vi "Header data_MClr.vi"(0 "base path":path=path "C:/", 1 "prompt (Create Folder)":string="logsController", 2 "file name":string, 5 "Error In":errorcluster) -> (14 "refnum out":refnum<file>, 19 "error out":errorcluster)   [LabVIEW 2018]
uses:
  Global textParse.vi
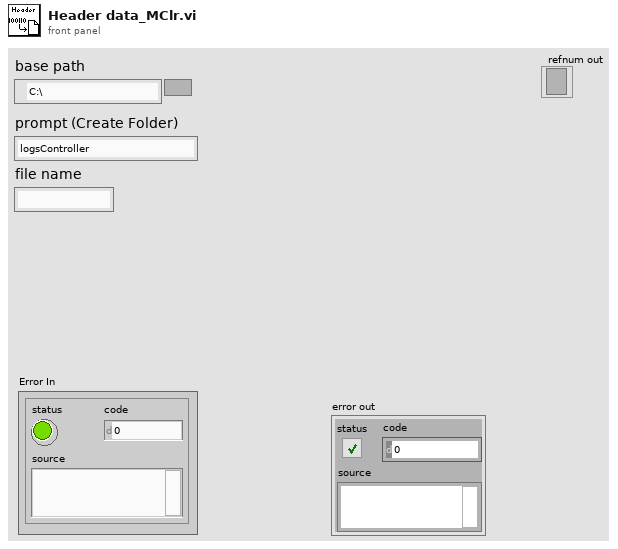
[diagram p1: front panel]
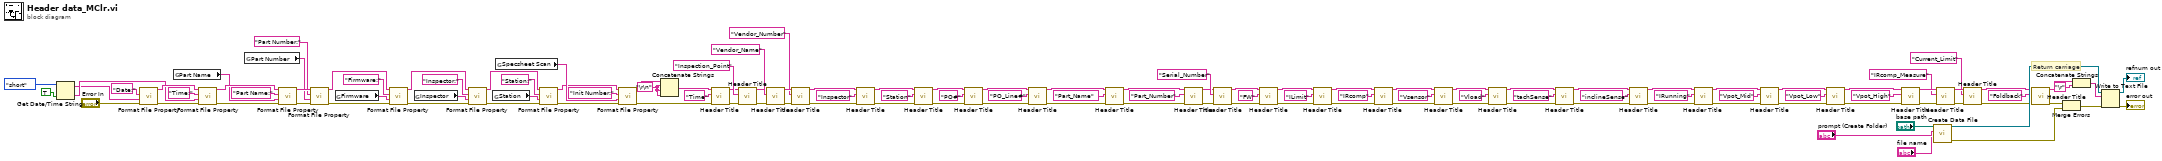
[diagram p0: block diagram]
diagram:
  w27 = "\r\n"
  # "Return carriage"
  n1 = Get Date/Time String(date format (0)=enum16{"short", "long", "abbreviated"}."short", want seconds? (F)=TRUE) -> (date string=w40:string, time string=w41:string)  [unwired: 1 in]
  n2 = call "Format File Property.vi"("Error In"="Error In", "File Property Value"=w40, "File Property Name"="Date:") -> ("Error Out"=w47:errorcluster, "String out"=w46:string)  [unwired: 7 in]
  n3 = global read "Global textParse.vi" "Part Name"() -> (w36:string)
  n4 = call "Format File Property.vi"("Error In"=w47, "File Property Value"=w41, "File Property Name"="Time:", "String in"=w46) -> ("Error Out"=w44:errorcluster, "String out"=w45:string)  [unwired: 6 in]
  n5 = global read "Global textParse.vi" "Part Number"() -> (w35:string)
  n6 = call "Format File Property.vi"("Error In"=w44, "File Property Value"=w36, "File Property Name"="Part Name:", "String in"=w45) -> ("Error Out"=w42:errorcluster, "String out"=w43:string)  [unwired: 6 in]
  n7 = call "Format File Property.vi"("Error In"=w42, "File Property Value"=w35, "File Property Name"="Part Number:" ("File Property Value"), "String in"=w43) -> ("Error Out"=w18:errorcluster, "String out"=w21:string)  [unwired: 6 in]
  n8 = global read "Global textParse.vi" "Firmware"() -> (w19:string)
  n9 = call "Format File Property.vi"("Error In"=w18, "File Property Value"=w19, "File Property Name"="Firmware:", "String in"=w21) -> ("Error Out"=w14:errorcluster, "String out"=w15:string)  [unwired: 6 in]
  n10 = global read "Global textParse.vi" "Inspector"() -> (w10:string)
  n11 = call "Format File Property.vi"("Error In"=w14, "File Property Value"=w10, "File Property Name"="Inspector:", "String in"=w15) -> ("Error Out"=w17:errorcluster, "String out"=w16:string)  [unwired: 6 in]
  n12 = global read "Global textParse.vi" "Station"() -> (w11:string)
  n13 = global read "Global textParse.vi" "Specsheet Scan"() -> (w22:string)
  n14 = call "Format File Property.vi"("Error In"=w17, "File Property Value"=w11, "File Property Name"="Station:", "String in"=w16) -> ("Error Out"=w8:errorcluster, "String out"=w9:string)  [unwired: 6 in]
  n15 = call "Format File Property.vi"("Error In"=w8, "File Property Value"=w22, "File Property Name"="Init Number:", "String in"=w9) -> ("Error Out"=w4:errorcluster, "String out"=w28:string)  [unwired: 6 in]
  n16 = Concatenate Strings(w28, w27, w27, w27) -> (w5:string)
  n17 = call "Header Title.vi"("Error In"=w4, "Header Title"="Time", "String in"=w5) -> ("Error Out"=w7:errorcluster, "String out"=w6:string)  [unwired: 7 in]
  n18 = call "Header Title.vi"("Error In"=w7, "Header Title"="Inspection_Point", "String in"=w6) -> ("Error Out"=w48:errorcluster, "String out"=w49:string)  [unwired: 7 in]
  n19 = call "Header Title.vi"("Error In"=w48, "Header Title"="Vendor_Name" ("File Property Name"), "String in"=w49) -> ("Error Out"=w60:errorcluster, "String out"=w68:string)  [unwired: 7 in]
  n20 = call "Header Title.vi"("Error In"=w60, "Header Title"="Vendor_Number" ("File Property Name"), "String in"=w68) -> ("Error Out"=w59:errorcluster, "String out"=w61:string)  [unwired: 7 in]
  n21 = call "Header Title.vi"("Error In"=w59, "Header Title"="Inspector" ("File Property Name"), "String in"=w61) -> ("Error Out"=w58:errorcluster, "String out"=w64:string)  [unwired: 7 in]
  n22 = call "Header Title.vi"("Error In"=w58, "Header Title"="Station" ("File Property Name"), "String in"=w64) -> ("Error Out"=w57:errorcluster, "String out"=w63:string)  [unwired: 7 in]
  n23 = call "Header Title.vi"("Error In"=w57, "Header Title"="PO#" ("File Property Name"), "String in"=w63) -> ("Error Out"=w33:errorcluster, "String out"=w32:string)  [unwired: 7 in]
  n24 = call "Header Title.vi"("Error In"=w33, "Header Title"="PO_Line#", "String in"=w32) -> ("Error Out"=w30:errorcluster, "String out"=w31:string)  [unwired: 7 in]
  n25 = call "Header Title.vi"("Error In"=w30, "Header Title"="Part_Name" ("File Property Name"), "String in"=w31) -> ("Error Out"=w51:errorcluster, "String out"=w55:string)  [unwired: 7 in]
  n26 = call "Header Title.vi"("Error In"=w51, "Header Title"="Part_Number" ("File Property Name"), "String in"=w55) -> ("Error Out"=w52:errorcluster, "String out"=w53:string)  [unwired: 7 in]
  n27 = call "Header Title.vi"("Error In"=w52, "Header Title"="Serial_Number" ("string"), "String in"=w53) -> ("Error Out"=w79:errorcluster, "String out"=w78:string)  [unwired: 7 in]
  n28 = call "Header Title.vi"("Error In"=w79, "Header Title"="FW", "String in"=w78) -> ("Error Out"=w86:errorcluster, "String out"=w85:string)  [unwired: 7 in]
  n29 = call "Header Title.vi"("Error In"=w86, "Header Title"="ILimit", "String in"=w85) -> ("Error Out"=w84:errorcluster, "String out"=w83:string)  [unwired: 7 in]
  n30 = call "Header Title.vi"("Error In"=w84, "Header Title"="IRcomp", "String in"=w83) -> ("Error Out"=w76:errorcluster, "String out"=w77:string)  [unwired: 7 in]
  n31 = call "Header Title.vi"("Error In"=w76, "Header Title"="Vsensor" ("string"), "String in"=w77) -> ("Error Out"=w107:errorcluster, "String out"=w111:string)  [unwired: 7 in]
  n32 = call "Header Title.vi"("Error In"=w107, "Header Title"="Vload" ("string"), "String in"=w111) -> ("Error Out"=w95:errorcluster, "String out"=w110:string)  [unwired: 7 in]
  n33 = call "Header Title.vi"("Error In"=w95, "Header Title"="tachSense" ("string"), "String in"=w110) -> ("Error Out"=w91:errorcluster, "String out"=w94:string)  [unwired: 7 in]
  n34 = call "Header Title.vi"("Error In"=w91, "Header Title"="inclineSense", "String in"=w94) -> ("Error Out"=w92:errorcluster, "String out"=w93:string)  [unwired: 7 in]
  n35 = call "Header Title.vi"("Error In"=w92, "Header Title"="IRunning" ("Measured Data"), "String in"=w93) -> ("Error Out"=w90:errorcluster, "String out"=w109:string)  [unwired: 7 in]
  n36 = call "Header Title.vi"("Error In"=w90, "Header Title"="Vpot_Mid" ("Measured Data"), "String in"=w109) -> ("Error Out"=w87:errorcluster, "String out"=w88:string)  [unwired: 7 in]
  n37 = call "Header Title.vi"("Error In"=w87, "Header Title"="Vpot_Low", "String in"=w88) -> ("Error Out"=w102:errorcluster, "String out"=w105:string)  [unwired: 7 in]
  n38 = call "Header Title.vi"("Error In"=w102, "Header Title"="Vpot_High", "String in"=w105) -> ("Error Out"=w101:errorcluster, "String out"=w104:string)  [unwired: 7 in]
  n39 = call "Create Data File.vi"("file name"="file name", "prompt (Create Folder)"="prompt (Create Folder)", "base path"="base path") -> ("Error Out"=w120:errorcluster, "File Refnum"=w122:refnum<file>)  [unwired: 7 in]
  n40 = call "Header Title.vi"("Error In"=w101, "Header Title"="IRcomp_Measure", "String in"=w104) -> ("Error Out"=w100:errorcluster, "String out"=w103:string)  [unwired: 7 in]
  n41 = call "Header Title.vi"("Error In"=w100, "Header Title"="Current_Limit", "String in"=w103) -> ("Error Out"=w1:errorcluster, "String out"=w2:string)  [unwired: 7 in]
  n42 = call "Header Title.vi"("Error In"=w1, "Header Title"="Foldback", "String in"=w2) -> ("Error Out"=w74:errorcluster, "String out"=w75:string)  [unwired: 7 in]
  n43 = Merge Errors(w74, w120) -> (w121:errorcluster)
  n44 = Concatenate Strings(w75, "\r") -> (w106:string)
  n45 = Write to Text File(file (use dialog)=w122, text=w106, error in=w121) -> (refnum out=→"refnum out":refnum<file>, error out=→"error out":errorcluster)  [unwired: 1 in, 1 out]
